vi "user interface page 2.vi"() -> ()   [LabVIEW 2023]
panel:
  out "DDD":bool
  out "TDM":bool
  out "TCS":bool
  out "CAN BUS":bool
  # "HEALTH STATUS"
  # "Failure list for Malfunction Data"
  # "No."
  # "Short fail. description"
  # "Operation hint"
  # "80"
  # "data recorder failure"
  # "repair as soon as possible"
  # "Scroll"
  # "Up"
  # "Down"
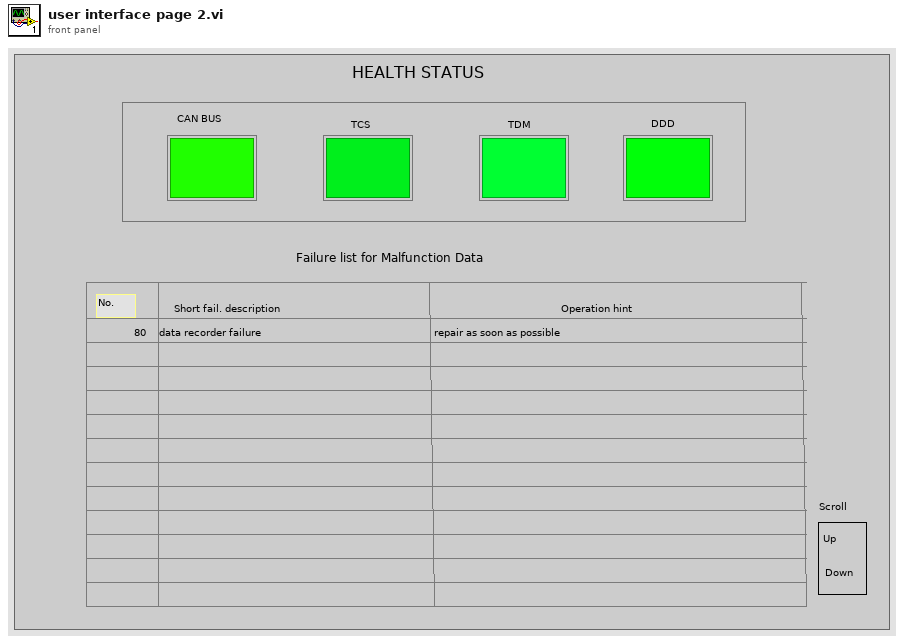
[diagram p1: front panel]
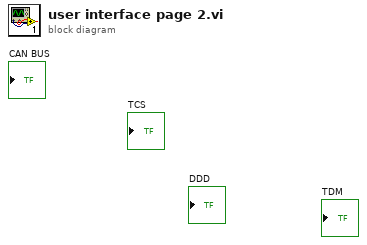
[diagram p0: block diagram]
diagram:
